vi "Ball Detection.vi"(1 "Camera Settings":T3={"fps"=15, "compression"=5, "Image Size"=enum."320x240"}) -> (0 "Ball Target":T1)   [LabVIEW 2013]
uses:
  <vilib>/Rock Robotics/WPI/Camera/WPI_CameraSettings Read MJPG.ctl
  <vilib>/Rock Robotics/WPI/Camera/WPI_CameraImageSize.ctl
  <resource>/objmgr/IMAQImage.rc
panel:
  in  "Targets":i32=3
  in  "Area Size Limit %":dbl=0.4 format="%#_13g"
  in  "Instructions:":string="Use the tab immediately below to choose the image source. Update the camera settings or the image directory so that you have images or video to test with.\n\nCalibration:\nYou can update Color Component ranges directly, or by clicking and drawing a line across the upper third of a ball within the image -- example shown below-right.\n\nUse Debugging tab to view intermediate results. Adjust Std Dev multipliers and line to achieve the desired HSV upper and lower threshold limits.\n\nArea Size LImit is used to ignore objects too small or balls too far away to care about.\n\nTargets identifies how many of the top scores to return.\n\nThe Details tab contains center, radius, and score details of each object."
  out "loop time ms":u32
  in  "Score Cutoff":dbl(slide)=70.58823529411765 scale=0.0..100.0
  in  "Color Components":T2={"Hue"={243.23333311080933, 20.233333110809326}, "Sat"={125.60287475585938, 242.93045043945312}, "Val"={83.88507843017578, 225.38158416748047}} {"Val" scale=0.0..255.0; "Sat" scale=0.0..255.0; "Hue" scale=0.0..255.0 scale format="%#_3g"}
  out "Error":bool
  in  "Image Source":enum32{"Files", "Camera"}(tab)=enum."Camera"
  in  "List of image files":i32(listbox)
  in  "Image Directory":path=path "2014 Vision Target"
  in  "Tabbed Info":enum32{"Debugging", "Details"}(tab)
  in  "Annotations":enum16{"None", "Good", "All"}(ring)=enum."Good"
  out "Initial Mask":T5(plugin-control)
  out "Fitted Mask":T5(plugin-control)
  out "Ranked Objects":T6(array[cluster]) {"Score" format="%#.1g"}
  out "Image":T5(plugin-control)
  # "Ranking Colors:\n1. green\n2. cyan\n3. magenta\n4. orange"
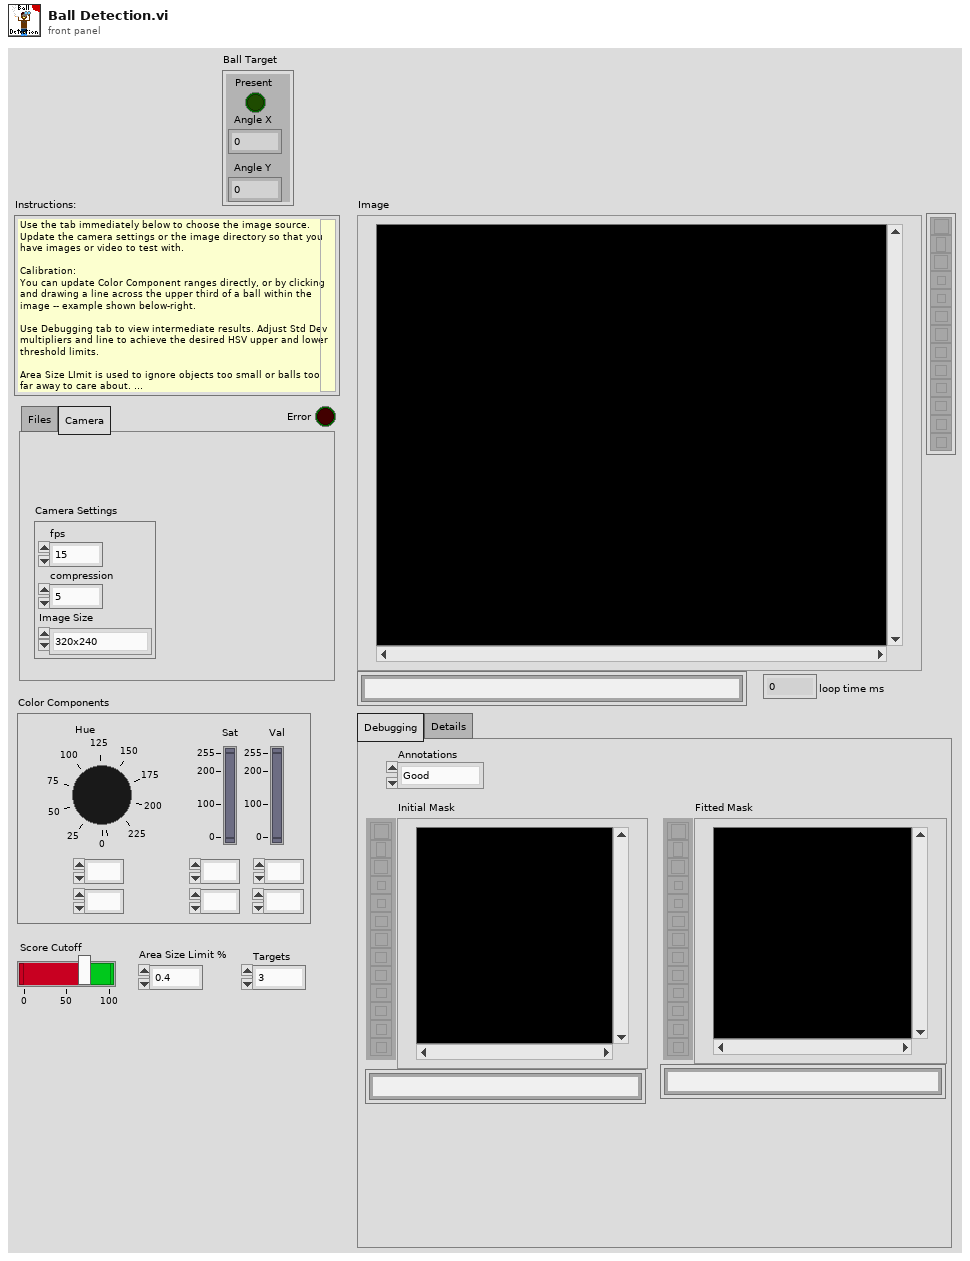
[diagram p1: front panel]
types:
  T1 = cluster{"Present":bool, "Angle X":dbl, "Angle Y":dbl}
  T2 = cluster{"Hue":cluster{dbl, dbl}, "Sat":cluster{dbl, dbl}, "Val":cluster{dbl, dbl}}
  T3 = typedef "WPI_CameraSettings Read MJPG.ctl" = cluster{"fps":i32, "compression":i32, "Image Size":T4}
  T4 = typedef "WPI_CameraImageSize.ctl" = enum16{"640x480", "320x240", "160x120"}
  T5 = typedef "IMAQ Image.ctl" = refnum<image>
  T6 = cluster{"Score":sgl, "Fitted Circle":cluster{"Center":cluster{"X":sgl, "Y":sgl}, "Radius":dbl, "Circle Rect":cluster{"L":sgl, "T":sgl, "R":sgl, "B":sgl}, "Roundness":dbl, "SNR (dB)":dbl}, "Search Rect":cluster{"L":sgl, "T":sgl, "R":sgl, "B":sgl}, "Details":cluster{"Edge":sgl, "Area":sgl, "Circ":sgl, "Diam":sgl}}[]
  T7 = typedef "Image Type" = u32
  T8 = cluster{"Circle Found":bool, "Fitted Circle":cluster{"Center":cluster{"X":sgl, "Y":sgl}, "Radius":dbl, "Center":cluster{"X":sgl, "Y":sgl}, "Radius":dbl, "Roundness":dbl, "Strength":dbl, "SNR (dB)":dbl}, "Array":dbl[], "Sorted Data":dbl[][]}[]
  T9 = cluster{"Score":dbl, "Fitted Circle":cluster{"Center (Pixels)":cluster{"X":sgl, "Y":sgl}, "Radius (Pixels)":dbl, "Circle Rect":cluster{"Left":sgl, "Top":sgl, "Right":sgl, "Bottom":sgl}, "Roundness (RW)":dbl, "Average SNR (dB)":dbl}, "Search Rect":cluster{"Left":sgl, "Top":sgl, "Right":sgl, "Bottom":sgl}, "Details":cluster{"Edges":sgl, "Circ/Rect":sgl, "Diam/Diam":sgl, "Circularity":sgl}}[]
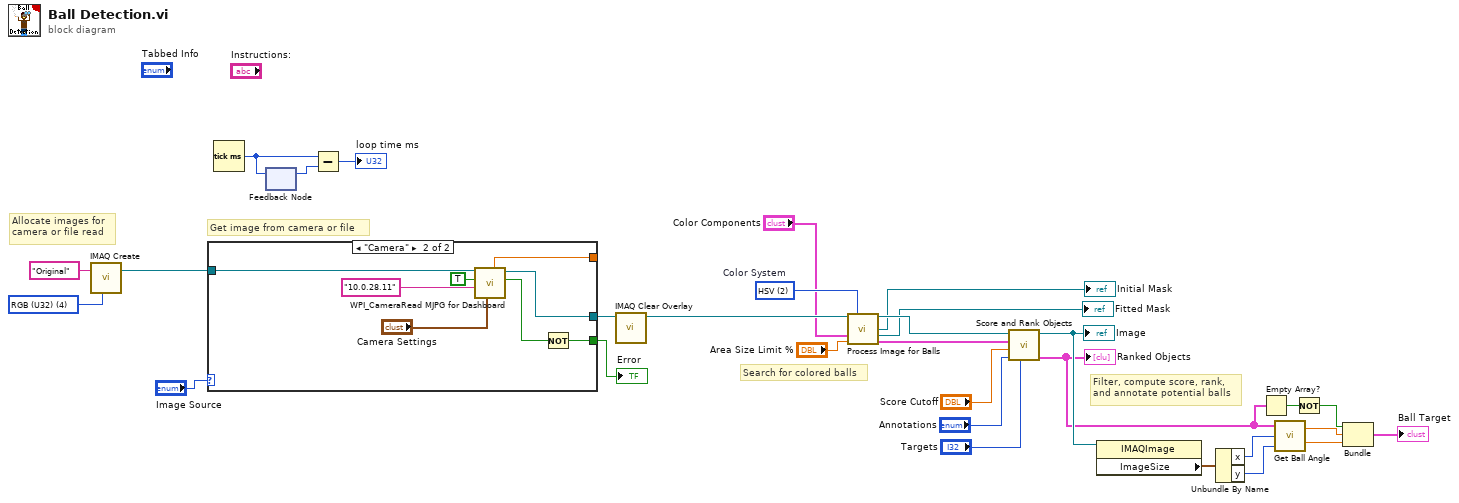
[diagram p0: block diagram]
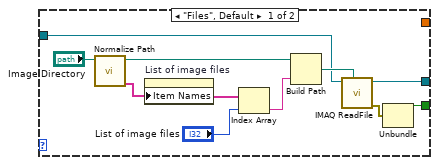
[diagram p2: hidden frame]
diagram:
  w12 = u16 2 items=["RGB", "HSL", "HSV", "HSI"]  # Color System
  w30 = T7 4 items=["Grayscale (U8)", "Grayscale (I16)", "Grayscale (SGL)", "Complex (CSG)", "RGB (U32)", "HSL (U32)", "RGB (U64)", "Grayscale (U16)"] ("Image Type")
  # "Search for colored balls"
  # "Filter, compute score, rank,\nand annotate potential balls"
  # "Get image from camera or file"
  # "Allocate images for\ncamera or file read"
  n1 = call "IMAQ Create"("Image Name"="Original", "Image Type"=w30) -> ("New Image"=w28:T5)  [unwired: 3 in, 1 out]
  n2 = case shown="\"Camera\"" "Image Source" {
    tunnel: [w37 w47] -> w27
    tunnel: w28 -> [w36 w48]
    tunnel: [w34 w43] -> w25
    tunnel: [_ w42] -> _
    frame "Files", Default {
      n3 = call "Normalize Path.vi"("Image Directory"="Image Directory") -> ("Filenames"=w33:string[], "Path"=w31:path)  [unwired: 9 in]
      n4 = property on="List of image files" class="LstBox (strict)"("Item Names"=w33) -> ()  [unwired: 2 in, 2 out]
      n5 = Index Array(array=w33, index="List of image files") -> (element=w39:string)
      n6 = Build Path(base path=w31, name or relative path=w39) -> (appended path=w38:path)
      n7 = call "IMAQ ReadFile"("File Path"=w38, "Image"=w36) -> ("error out"=w35:errorcluster, "Image Out"=w37:T5)  [unwired: 5 in, 3 out]
      n8 = Unbundle(w35) -> ("status"=w34:bool)  [unwired: 2 out]
    }
    frame "Camera" {
      n9 = call <vilib>:"WPI_CameraRead MJPG for Dashboard.vi"("Camera Settings"="Camera Settings", "Camera IP"="10.0.28.11", "Enable"=TRUE, "Refnum in"=w48) -> ("Active"=w45:bool, "Refnum out"=w47:T5, "Bandwidth (Mbps)"=w42:dbl)  [unwired: 4 in, 1 out]
      n10 = Not(x=w45) -> (.not. x?=w43:bool)
    }
  }
  "Error" <- w25
  n11 = Tick Count (ms)() -> (millisecond timer value=w24:u32)
  n12 = feedback #1() -> (w23:u32)  [unwired: 1 in]
  n13 = feedback-in #1(w24) -> ()
  n14 = Subtract(x=w24, y=w23) -> (x-y=→"loop time ms":u32)
  n15 = call "IMAQ Clear Overlay"("Image"=w27) -> ("Image Out"=w19:T5)  [unwired: 9 in, 1 out]
  n16 = call "Process Image for Balls.vi"("Src Image"=w19, "Color Mode 2"=w12, "Color"="Color Components", "Area Cutoff %"="Area Size Limit %") -> ("Src Image Out"=w17:T5, "First Threshold"=→"Initial Mask":T5, "Fitted"=→"Fitted Mask":T5, "Potential"=w16:T8)  [unwired: 8 in]
  n17 = call "Score and Rank Objects.vi"("Targets"="Targets", "Annotations"="Annotations", "Score Limit"="Score Cutoff", "Object Info"=w16, "Image in"=w17) -> ("Object Info"=w4:T9, "Annotated Image"=w10:T5)  [unwired: 5 in]
  "Image" <- w10
  "Ranked Objects" <- w4
  n18 = property class="IMAQImage"(reference=w10) -> ("ImageSize"=w9:cluster{"x":i32, "y":i32})  [unwired: 1 in, 2 out]
  n19 = Unbundle By Name(w9) -> ("x"=w8:i32, "y"=w7:i32)
  n20 = Empty Array?(array=w4) -> (empty?=w3:bool)
  n21 = call "Get Ball Angle.vi"("Camera Res Y"=w7, "Camera Res X"=w8, "Ranked Objects"=w4) -> ("Angle Y"=w5:dbl, "Angle X"=w6:dbl)
  n22 = Not(x=w3) -> (.not. x?=w2:bool)
  n23 = Bundle(w2, "Angle X"=w6, "Angle Y"=w5) -> (→"Ball Target":cluster{bool, "Angle X":dbl, "Angle Y":dbl})  [unwired: 1 in]
